vi "N6705b_Emulating_Mode_Setting.vi"(8 "error in (no error)":errorcluster {"code" format="%.0x"}, 10 "Mode":T1(ring), 11 "VISA resource name":refnum<visa-resource-name>) -> (0 "error out":errorcluster {"code" format="%.0x"}, 3 "VISA resource name out":refnum<visa-resource-name>)   [LabVIEW 2015]
uses:
  <instrlib>/Agilent N6700 Series/Agilent N6700 Series.lvlib
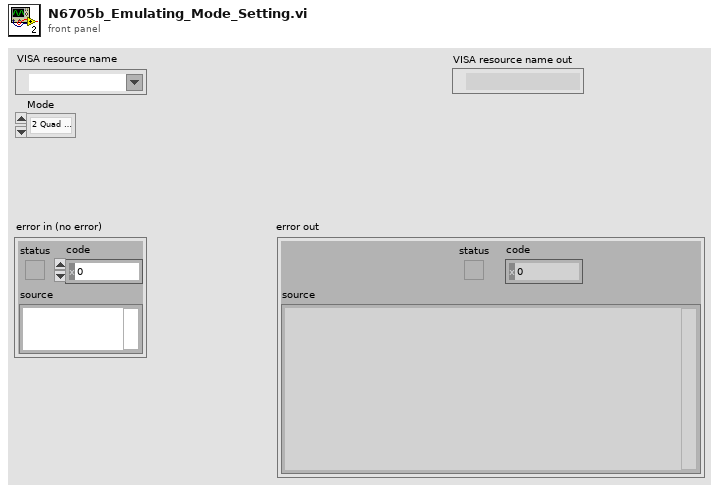
[diagram p1: front panel]
types:
  T1 = enum16{"2 Quad Power Supply", "Unipower Supply", "CC Load", "CV Load", "VM", "CM"}
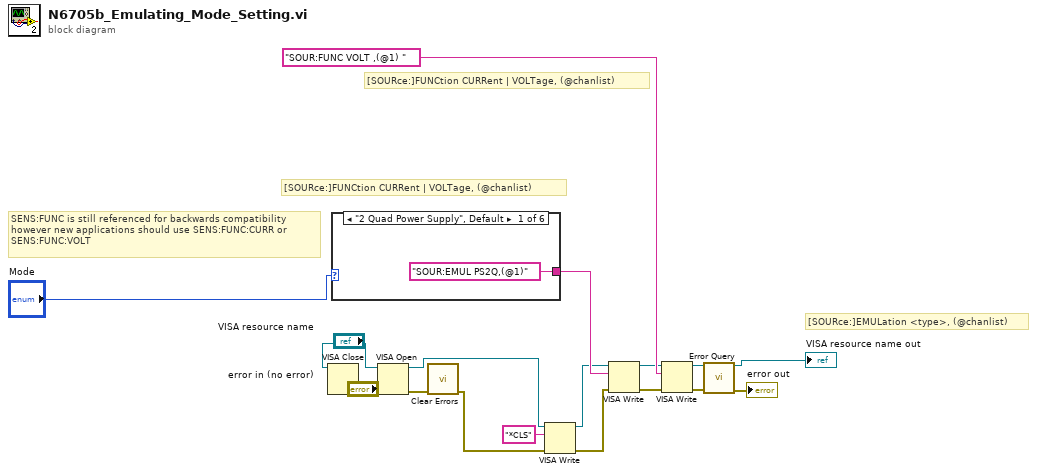
[diagram p0: block diagram]
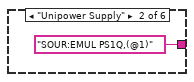
[diagram p2: hidden frame]
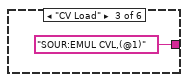
[diagram p3: hidden frame]
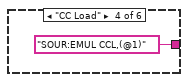
[diagram p4: hidden frame]
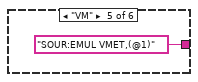
[diagram p5: hidden frame]
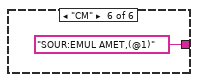
[diagram p6: hidden frame]
diagram:
  # "[SOURce:]FUNCtion CURRent | VOLTage, (@chanlist)"
  # "[SOURce:]FUNCtion CURRent | VOLTage, (@chanlist)"
  # "[SOURce:]EMULation <type>, (@chanlist)"
  # "SENS:FUNC is still referenced for backwards compatibility\nhowever new applications should use SENS:FUNC:CURR or\nSENS:FUNC:VOLT"
  n1 = VISA Close(VISA resource name="VISA resource name", error in (no error)="error in (no error)") -> (error out=w13:errorcluster)
  n2 = case shown="\"2 Quad Power Supply\", Default" "Mode" {
    tunnel: ["SOUR:EMUL PS2Q,(@1)" ("write buffer") "SOUR:EMUL PS1Q,(@1)" ("write buffer") "SOUR:EMUL CVL,(@1)" ("write buffer") "SOUR:EMUL CCL,(@1)" ("write buffer") "SOUR:EMUL VMET,(@1)" ("write buffer") "SOUR:EMUL AMET,(@1)" ("write buffer")] -> w11
    frame "2 Quad Power Supply", Default {
    }
    frame "Unipower Supply" {
    }
    frame "CV Load" {
    }
    frame "CC Load" {
    }
    frame "VM" {
    }
    frame "CM" {
    }
  }
  n3 = VISA Open(error in (no error)=w13, VISA resource name="VISA resource name") -> (VISA resource name=w2:refnum<visa-resource-name>, error out=w16:errorcluster)  [unwired: 3 in]
  n4 = call <vilib>:"Clear Errors.vi"("error in (no error)"=w16) -> ("error out"=w1:errorcluster)  [unwired: 5 in, 1 out]
  n5 = VISA Write(VISA resource name=w2, write buffer="*CLS", error in (no error)=w1) -> (VISA resource name out=w4:refnum<visa-resource-name>, error out=w3:errorcluster)  [unwired: 1 out]
  n6 = VISA Write(VISA resource name=w4, write buffer=w11, error in (no error)=w3) -> (VISA resource name out=w9:refnum<visa-resource-name>, error out=w7:errorcluster)  [unwired: 1 out]
  n7 = VISA Write(VISA resource name=w9, write buffer="SOUR:FUNC VOLT ,(@1) ", error in (no error)=w7) -> (VISA resource name out=w8:refnum<visa-resource-name>, error out=w6:errorcluster)  [unwired: 1 out]
  n8 = call <instrlib>:"Error Query.vi"("VISA resource name"=w8, "error in (no error)"=w6) -> ("VISA resource name out"=→"VISA resource name out":refnum<visa-resource-name>, "error out"=→"error out":errorcluster)  [unwired: 10 in, 2 out]
